vi "Get Global Attribute.vi"(8 "Error In":errorcluster, 11 "Name":string) -> (0 "Error Out":errorcluster, 2 "Found":bool, 3 "Value":variant)   [LabVIEW 2013, in "TS.lvlib"]
doc: "Reentrant."
uses:
  TS.lvlib
  Variant Global.vi
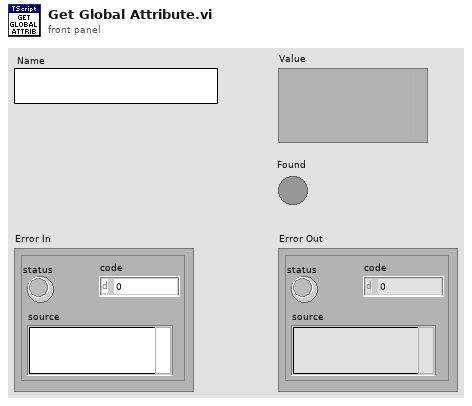
[diagram p1: front panel]
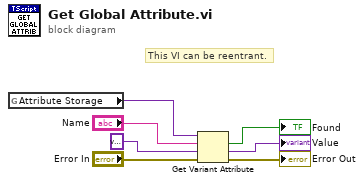
[diagram p0: block diagram]
diagram:
  # "This VI can be reentrant."
  n1 = global read "Variant Global.vi" "Attribute Storage"() -> (w7:variant)
  n2 = Get Variant Attribute(Variant=w7, name="Name", default value (empty Variant)=variant ("Value"), error in="Error In") -> (found=→"Found":bool, value=→"Value":variant, error out=→"Error Out":errorcluster)  [unwired: 1 out]
